vi "Indicator Test.vi"() -> ()   [LabVIEW 2011, in "LVH-Xbox-One-Controller.lvlib"]
uses:
  Private/Type Defs/Indicators/Controller.ctl
  Private/Type Defs/Indicators/A.ctl
  Private/Type Defs/Indicators/B.ctl
  Private/Type Defs/Indicators/X.ctl
  Private/Type Defs/Indicators/Y.ctl
  Private/Type Defs/Indicators/Left Bumper.ctl
  Private/Type Defs/Indicators/Right Bumper.ctl
  Private/Type Defs/Indicators/View.ctl
  Private/Type Defs/Indicators/Menu.ctl
  Private/Type Defs/Indicators/Thumbstick_Analog.ctl
  Private/Type Defs/Indicators/Slider.ctl
  Private/Type Defs/Indicators/DPad.ctl
  Private/Type Defs/Indicators/DPad Enum.ctl
  <vilib>/Utility/inputDevices.llb/closeJoystick.vi
  <vilib>/Utility/inputDevices.llb/joystickAcquire.vi
  LVH-Xbox-One-Controller.lvlib
panel:
  out "Controller":T1={"A Button"=FALSE, "B Button"=FALSE, "X Button"=FALSE, "Y Button"=FALSE, "Left Bumper"=FALSE, "Right Bumper"=FALSE, "View Button"=FALSE, "Menu Button"=FALSE, "Left Stick"={[], []}, "Right Stick"={[], []}, "Trigger"=0, "D-Pad"=5} {"Trigger" scale=32767.0..-32768.0}
  in  "Stop Button":bool
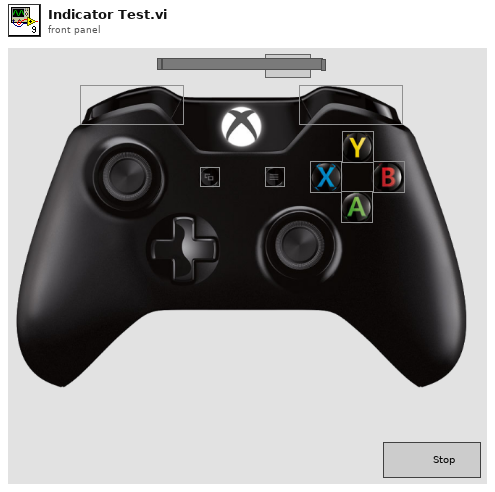
[diagram p1: front panel]
types:
  T1 = typedef "LVH-Xbox-One-Controller.lvlib/Controller.ctl" = cluster{"A Button":T2, "B Button":T3, "X Button":T4, "Y Button":T5, "Left Bumper":T6, "Right Bumper":T7, "View Button":T8, "Menu Button":T9, "Left Stick":T10, "Right Stick":T10, "Trigger":T11, "D-Pad":T12}
  T2 = typedef "LVH-Xbox-One-Controller.lvlib/A.ctl" = bool
  T3 = typedef "LVH-Xbox-One-Controller.lvlib/B.ctl" = bool
  T4 = typedef "LVH-Xbox-One-Controller.lvlib/X.ctl" = bool
  T5 = typedef "LVH-Xbox-One-Controller.lvlib/Y.ctl" = bool
  T6 = typedef "LVH-Xbox-One-Controller.lvlib/Left Bumper.ctl" = bool
  T7 = typedef "LVH-Xbox-One-Controller.lvlib/Right Bumper.ctl" = bool
  T8 = typedef "LVH-Xbox-One-Controller.lvlib/View.ctl" = bool
  T9 = typedef "LVH-Xbox-One-Controller.lvlib/Menu.ctl" = bool
  T10 = typedef "LVH-Xbox-One-Controller.lvlib/Thumbstick_Analog.ctl" = cluster{i32[], i32[]}
  T11 = typedef "LVH-Xbox-One-Controller.lvlib/Slider.ctl" = i32
  T12 = typedef "LVH-Xbox-One-Controller.lvlib/DPad.ctl" = u16
  T13 = typedef "LVH-Xbox-One-Controller.lvlib/DPad Enum.ctl" = enum16{"Idle", "Up", "Up / Right", "Right", "Down / Right", "Down", "Down / Left", "Left", "Up / Left"}
  T14 = cluster{"X axis":i32, "Y axis":i32, "Z axis":i32, "X axis rotation":i32, "Y axis rotation":i32, "Z axis rotation":i32, "U axis":i32, "V axis":i32}
  T15 = cluster{"button 1":bool, "button 2":bool, "button 3":bool, "button 4":bool, "button 5":bool, "button 6":bool, "button 7":bool, "button 8":bool, "button 9":bool, "button 10":bool, "button 11":bool, "button 12":bool, "button 13":bool, "button 14":bool, "button 15":bool, "button 16":bool, "button 17":bool, "button 18":bool, "button 19":bool, "button 20":bool, "button 21":bool, "button 22":bool, "button 23":bool, "button 24":bool, "button 25":bool, "button 26":bool, "button 27":bool, "button 28":bool, "button 29":bool, "button 30":bool, "button 31":bool, "button 32":bool}
  T16 = cluster{"pov 1":i32, "pov 2":i32, "pov 3":i32, "pov 4":i32}
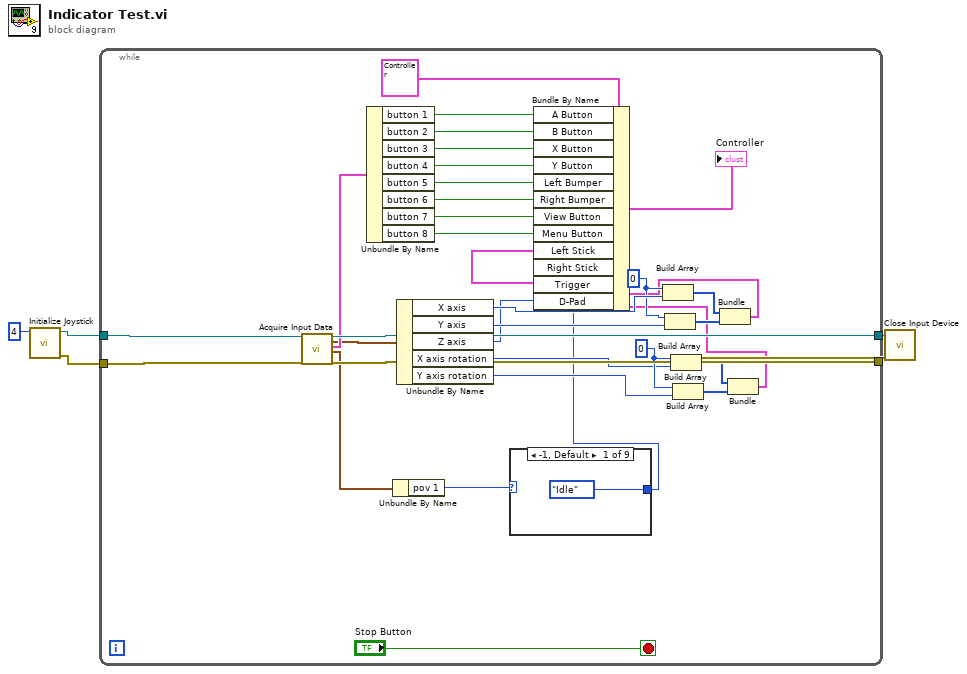
[diagram p0: block diagram]
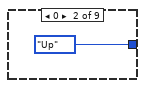
[diagram p2: hidden frame]
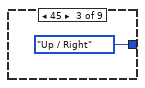
[diagram p3: hidden frame]
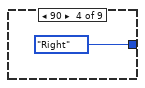
[diagram p4: hidden frame]
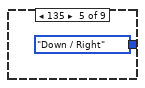
[diagram p5: hidden frame]
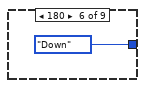
[diagram p6: hidden frame]
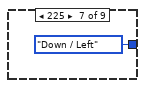
[diagram p7: hidden frame]
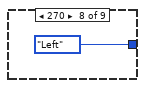
[diagram p8: hidden frame]
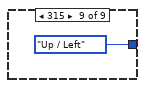
[diagram p9: hidden frame]
diagram:
  n1 = call <vilib>:"Initialize Joystick.vi"("device index"=4) -> ("error out"=w3:errorcluster, "device ID"=w2:refnum<k1>)  [unwired: 9 in]
  n2 = while {
    tunnel: [w38] -> w5
    tunnel: [w37] -> w4
    tunnel: w3 -> [w36]
    tunnel: w2 -> [w35]
    stop <- "Stop Button" stop-if-true
    w25 = 0 ("element")
    w28 = 0 ("element")
    n3 = call-poly <vilib>:"Acquire Input Data.vi"("device ID"=w35, "error in (no error)"=w36) -> ("device ID"=w38:refnum<k1>, "axis info"=w32:T14, "button info"=w33:T15, "direction info"=w8:T16, "error out"=w37:errorcluster)  [unwired: 13 in]
    n4 = Unbundle By Name(w33) -> ("button 1"=w20:bool, "button 2"=w19:bool, "button 3"=w18:bool, "button 4"=w17:bool, "button 5"=w16:bool, "button 6"=w15:bool, "button 7"=w13:bool, "button 8"=w12:bool)
    n5 = Unbundle By Name(w8) -> ("pov 1"=w7:i32)
    n6 = Unbundle By Name(w32) -> ("X axis"=w31:i32, "Y axis"=w22:i32, "Z axis"=w9:i32, "X axis rotation"=w24:i32, "Y axis rotation"=w23:i32)
    n7 = case shown="-1, Default" w7 {
      tunnel: [DPad_Enum."Idle" ("D-Pad") DPad_Enum."Up" ("D-Pad") DPad_Enum."Up / Right" ("D-Pad") DPad_Enum."Right" ("D-Pad") DPad_Enum."Down / Right" ("D-Pad") DPad_Enum."Down" ("D-Pad") DPad_Enum."Down / Left" ("D-Pad") DPad_Enum."Left" ("D-Pad") DPad_Enum."Up / Left" ("D-Pad")] -> w6
      frame -1, Default {
      }
      frame 0 {
      }
      frame 45 {
      }
      frame 90 {
      }
      frame 135 {
      }
      frame 180 {
      }
      frame 225 {
      }
      frame 270 {
      }
      frame 315 {
      }
    }
    n8 = Build Array(w28, w31) -> (w30:i32[])
    n9 = Build Array(w28, w22) -> (w29:i32[])
    n10 = Build Array(w25, w24) -> (w26:i32[])
    n11 = Build Array(w25, w23) -> (w27:i32[])
    n12 = Bundle(w30, w29) -> (w10:cluster{i32[], i32[]})  [unwired: 1 in]
    n13 = Bundle(w26, w27) -> (w11:cluster{i32[], i32[]})  [unwired: 1 in]
    n14 = Bundle By Name(cluster=T1 {"A Button"=FALSE, "B Button"=FALSE, "X Button"=FALSE, "Y Button"=FALSE, "Left Bumper"=FALSE, "Right Bumper"=FALSE, "View Button"=FALSE, "Menu Button"=FALSE, "Left Stick"={[], []}, "Right Stick"={[], []}, "Trigger"=0, "D-Pad"=0} ("Controller"), "A Button"=w20, "B Button"=w19, "X Button"=w18, "Y Button"=w17, "Left Bumper"=w16, "Right Bumper"=w15, "View Button"=w13, "Menu Button"=w12, "Left Stick"=w10, "Right Stick"=w11, "Trigger"=w9, "D-Pad"=w6) -> (→"Controller":T1)
  }
  n15 = call-poly <vilib>:"Close Input Device.vi"("error in (no error)"=w4, "device ID"=w5) -> ()  [unwired: 8 in, 1 out]
